vi "view -- rename scan files -- insert timestamp.vi"() -> ()   [LabVIEW 2012]
uses:
  tfolder.ctl
  tfolder -- monotonic segment.ctl
  sweep file name.ctl
  file -- scan filename action.ctl
panel:
  in  "REPLACE ???":bool
  out "suffix":string[](array[string])
  out "sweep path array OUT":T1[](array[typedef])
  in  "tfolder IN":T2={"tfolder path"=path "/snowfall/Users/arcadi/Desktop/Ultrasound/Experiment/YBCO_4/Round1/Sweep12/June_2011/062511/221.16400K_300_3100_001_062511.dat", "9folder path"=path "/snowfall/Users/arcadi/Desktop/Ultrasound/Experiment/YBCO_4/Round1/Sweep12/June_2011/062511/221.16400K_300_3100_001_062511.dat", "tfolder  -  file array"=[], "from index array"=[], "timestamp array"=[]}
  out "Array NEW":string[](array[string])
  out "Array ORIGINAL":string[](array[string])
  in  "t folder path":path=path "E:/data/Ultrasound/Experiment/ProbeTest/Probe10/YBCO_5/sweep6/9w"
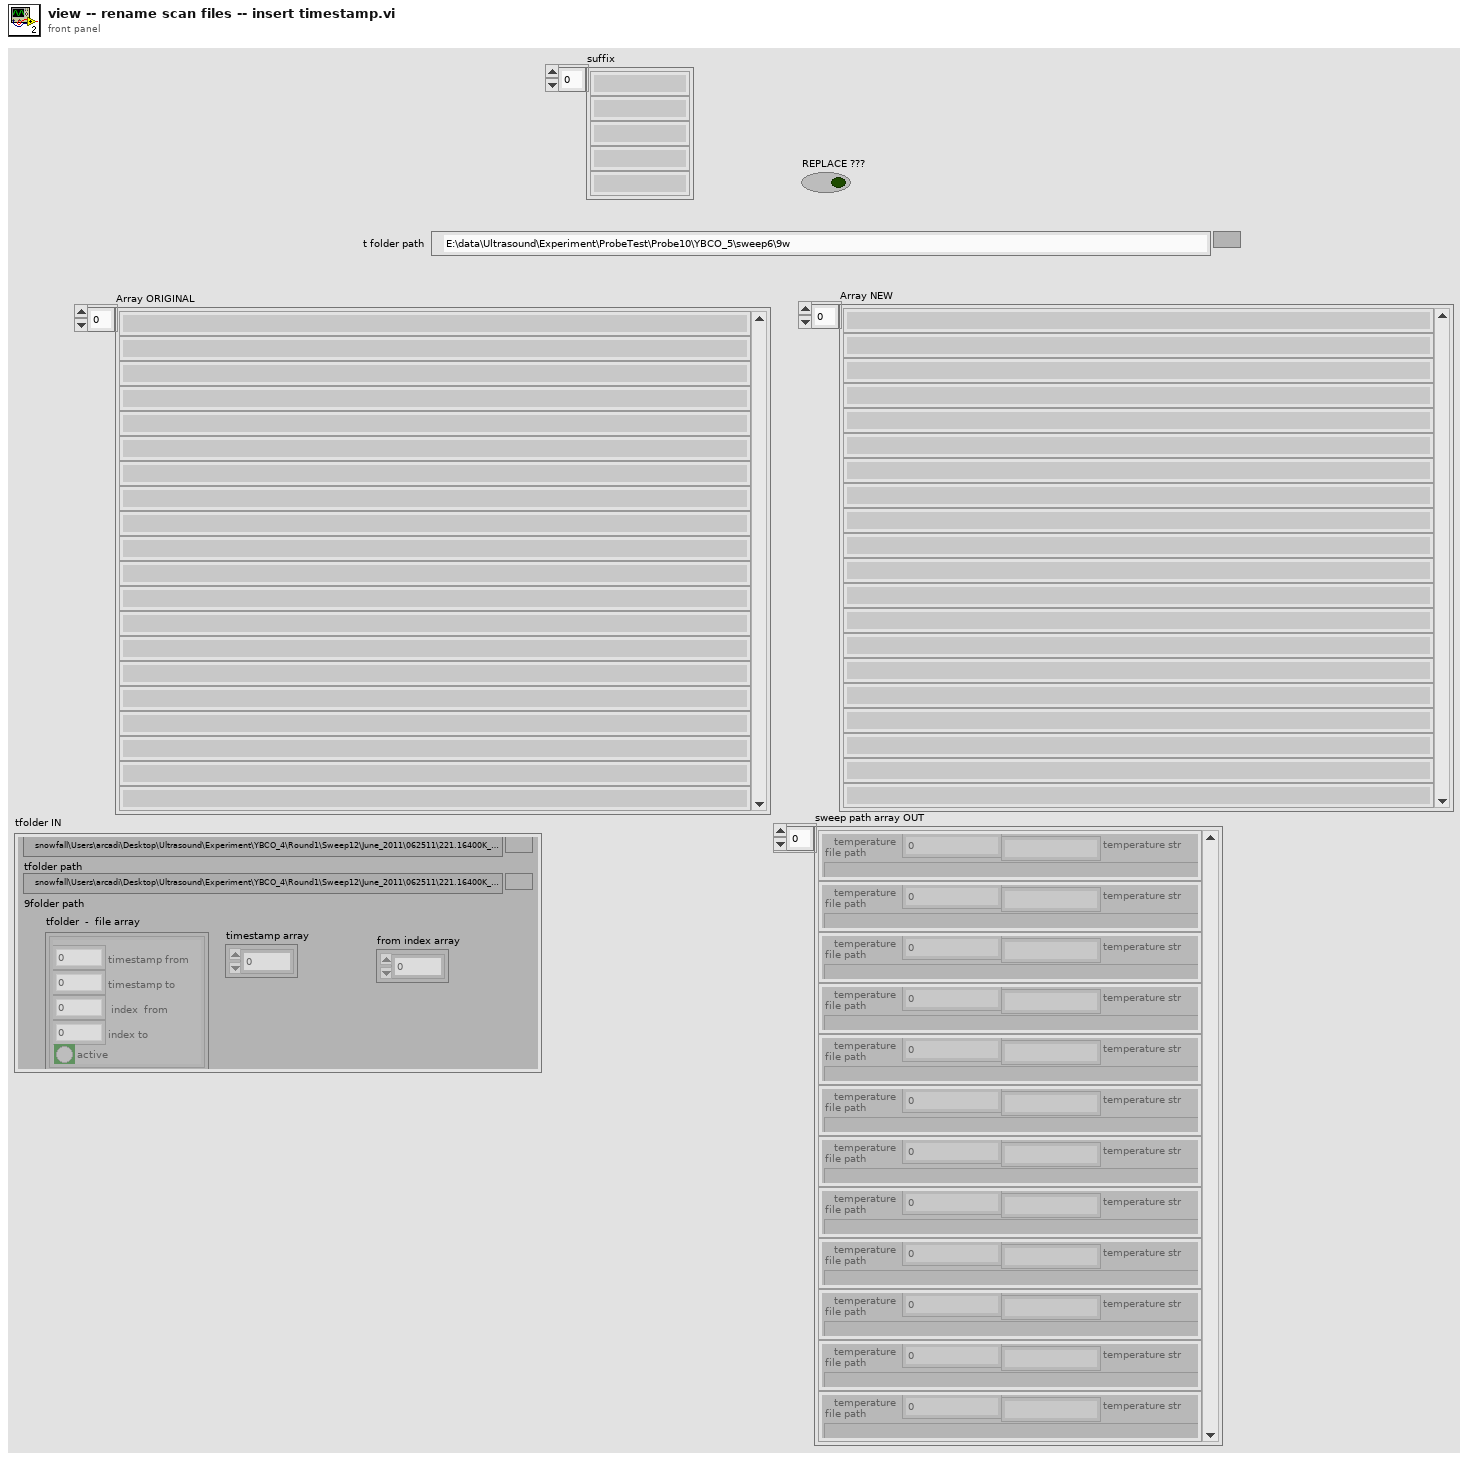
[diagram p1: front panel]
types:
  T1 = typedef "sweep file name.ctl" = cluster{"temperature":dbl, "temperature str":string, "file path":path, "last mod":timestamp, "file name str":string, "mod time(min)":dbl, "file format":enum16{"", "ascii", "binary"}}
  T2 = typedef "tfolder.ctl" = cluster{"tfolder path":path, "9folder path":path, "tfolder  -  file array":T3[], "from index array":i32[], "timestamp array":dbl[]}
  T3 = typedef "tfolder -- monotonic segment.ctl" = cluster{"timestamp from":dbl, "timestamp to":dbl, " index  from":i32, "index to":i32, "active":bool}
  T4 = enum16{"new", "update range", "update monotonic pieces", "init", "check", "reset", ""}
  T5 = typedef "file -- scan filename action.ctl" = enum16{"prefix base name", "datestring regexp", "parse datestring", "datestring", "filename regexp", "parse filename", "datestring regexp (no brackets)", "suffix base name"}
  T6 = typedef "file -- scan filename.ctl" = cluster{"mmddyy (str)":string, "counter (str)":string, "to F (kHz)":dbl, "from F (kHz)":dbl, "temperature (K)":dbl, "date/time string":string, "time stamp":timestamp, "base name":string, "temperature (str)":string, "from F (str)":string, "to F (str)":string, "format":enum16{"no date string", "with date string"}}
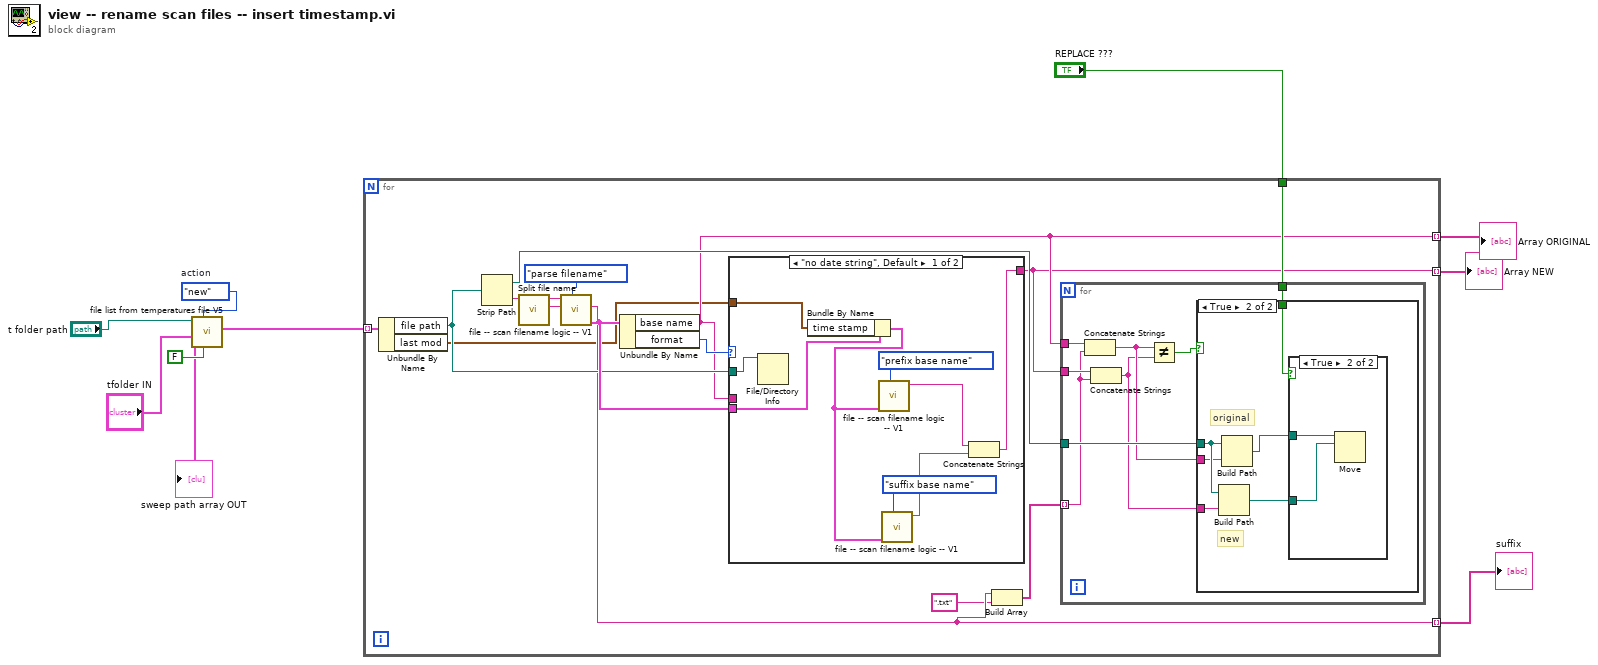
[diagram p0: block diagram]
diagram:
  w8 = T4."new"  # action
  n1 = call "file list from temperatures file V5.vi"("monotonic segments ON/OFF"=FALSE, "action"=w8, "tfolder IN"="tfolder IN", "tfolder file path  IN"="t folder path") -> ("sweep path array OUT"=w6:T1[])  [unwired: 3 in, 4 out]
  "sweep path array OUT" <- w6
  n2 = for {
    tunnel: w6 -> [w24] mode=indexing
    tunnel: [w13] -> w5 mode=indexing
    tunnel: [w12] -> w4 mode=indexing
    tunnel: [w15] -> w2 mode=indexing
    tunnel: "REPLACE ???" -> [w16]
    n3 = Unbundle By Name(w24) -> ("file path"=w18:path, "last mod"=w10:timestamp)
    n4 = Strip Path(path=w18) -> (stripped path=w17:path, name=w20:string)
    n5 = call "Split file name.vi"("file name"=w20) -> ("extension"=w15:string, "name"=w19:string)  [unwired: 8 in, 1 out]
    n6 = call "file -- scan filename logic -- V1.vi"("scan fileneme action"=file_--_scan_filename_action."parse filename", "base name IN"=w19) -> ("scan filename OUT"=w21:T6)  [unwired: 7 in, 2 out]
    n7 = Unbundle By Name(w21) -> ("base name"=w13:string, "format"=w22:enum16{"no date string", "with date string"})
    n8 = case shown="\"no date string\", Default" w22 {
      tunnel: [w45 w50] -> w12
      tunnel: w13 -> [_ w50]
      tunnel: w21 -> [w43 _]
      tunnel: w18 -> [w44 _]
      tunnel: w10 -> [w41 _]
      frame "no date string", Default {
        n9 = File/Directory Info(path=w44) -> ()  [unwired: 1 in, 7 out]
        n10 = Bundle By Name(cluster=w43, "time stamp"=w41) -> (w42:T6)
        n11 = call "file -- scan filename logic -- V1.vi"("scan fileneme action"=file_--_scan_filename_action."prefix base name", "scan filename IN"=w42) -> ("string OUT"=w47:string)  [unwired: 7 in, 2 out]
        n12 = call "file -- scan filename logic -- V1.vi"("scan fileneme action"=file_--_scan_filename_action."suffix base name", "scan filename IN"=w42) -> ("string OUT"=w46:string)  [unwired: 7 in, 2 out]
        n13 = Concatenate Strings(w47, w46) -> (w45:string)
      }
      frame "with date string" {
      }
    }
    n14 = Build Array(w15, ".txt") -> (w11:string[])
    n15 = for {
      tunnel: w17 -> [w32]
      tunnel: w16 -> [w28]
      tunnel: w13 -> [w27]
      tunnel: w12 -> [w26]
      tunnel: w11 -> [w25] mode=indexing
      n16 = Concatenate Strings(w27, w25) -> (w31:string)
      n17 = Concatenate Strings(w26, w25) -> (w30:string)
      n18 = Not Equal?(x=w31, y=w30) -> (x != y?=w29:bool)
      n19 = case shown="True" w29 {
        tunnel: w32 -> [_ w38]
        tunnel: w31 -> [_ w37]
        tunnel: w30 -> [_ w36]
        tunnel: w28 -> [_ w35]
        frame False {
        }
        frame True {
          # "new"
          # "original"
          n20 = Build Path(base path=w38, name or relative path=w36) -> (appended path=w33:path)
          n21 = Build Path(base path=w38, name or relative path=w37) -> (appended path=w34:path)
          n22 = case shown="True" w35 {
            tunnel: w34 -> [_ w40]
            tunnel: w33 -> [_ w39]
            frame False {
            }
            frame True {
              n23 = Move(source path=w40, 10:w39) -> ()  [unwired: 3 in, 3 out]
            }
          }
        }
      }
    }
  }
  "Array ORIGINAL" <- w5
  "Array NEW" <- w4
  "suffix" <- w2
